vi "VNA test.vi"() -> ()   [LabVIEW 2022 SP3, in "Agilent ENA Series.lvlib"]
uses:
  <instrlib>/Agilent ENA Series/Agilent ENA Series.lvlib
  <vilib>/Utility/file.llb/Write Delimited Spreadsheet (DBL).vi
panel:
  in  "Number of Measurement Points (201)":i32=201
  in  "file path (dialog if empty) 2":path
  out "source":string
  in  "Measurement Parameter (0:S11)":u16(ring) items=["S11", "S21", "S31", "S41", "S12", "S22", "S32", "S42", "S13", "S23", "S33", "S43", "S14", "S24", "S34", "S44", "A", "B", "C", "D", "R1", "R2", "R3", "R4", "AUX1", "AUX2", "TR", "T", "R"]
  out "Waveform Graph":dbl[](graph)
  in  "VISA resource name":refnum<visa-resource-name>
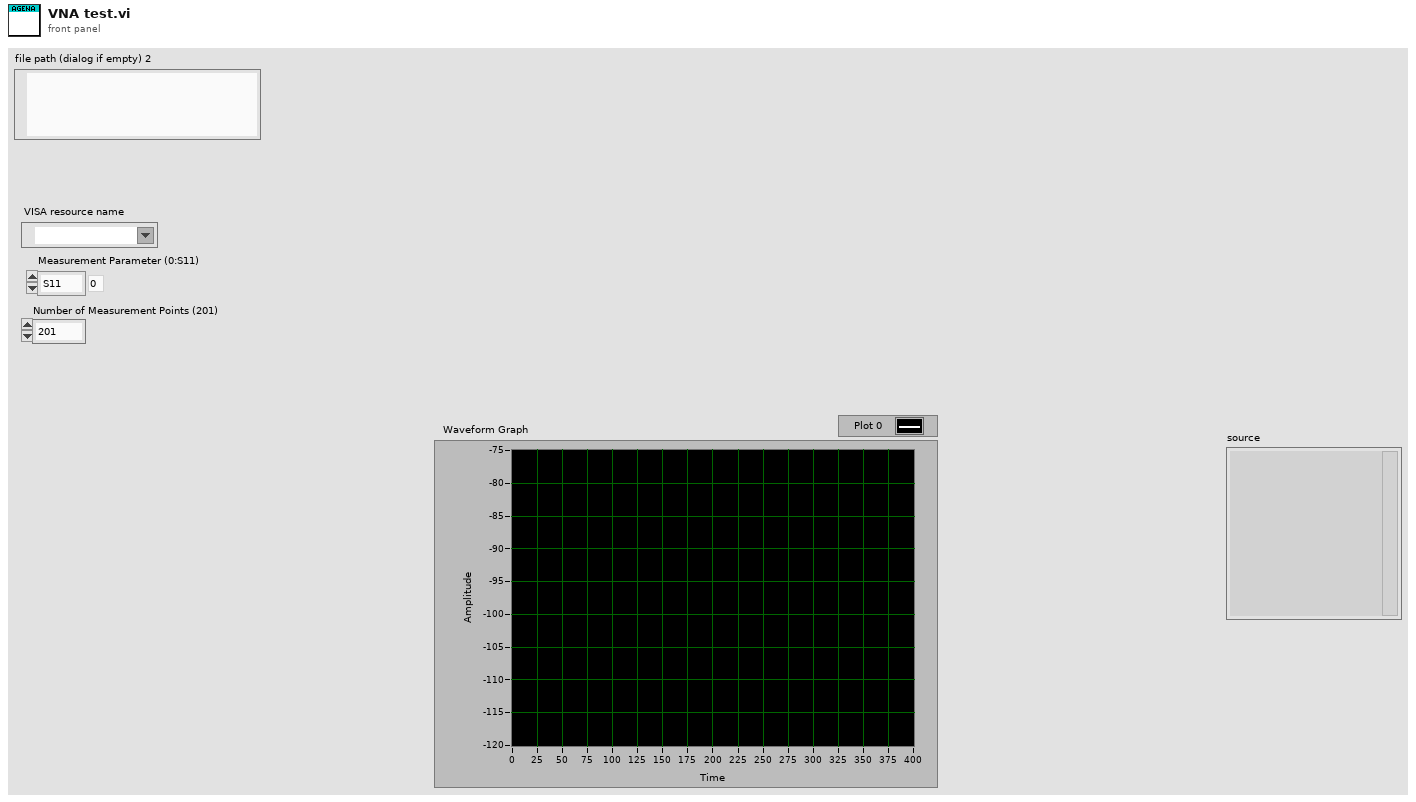
[diagram p1: front panel]
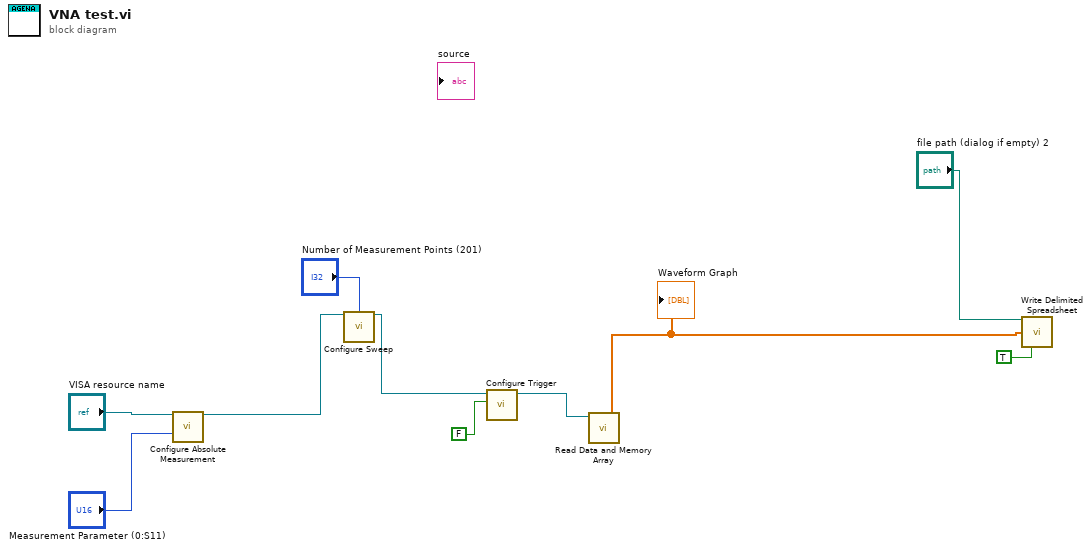
[diagram p0: block diagram]
diagram:
  n1 = call <instrlib>:"Configure Absolute Measurement.vi"("VISA resource name"="VISA resource name", "Measurement Parameter (0:S11)"="Measurement Parameter (0:S11)") -> ("VISA resource name out"=w3:refnum<visa-resource-name>)  [unwired: 12 in, 1 out]
  n2 = call <instrlib>:"Configure Sweep.vi"("VISA resource name"=w3, "Number of Measurement Points (201)"="Number of Measurement Points (201)") -> ("VISA resource name out"=w2:refnum<visa-resource-name>)  [unwired: 12 in, 1 out]
  n3 = call <instrlib>:"Configure Trigger.vi"("Continuous Sweep (T: Enable)"=FALSE, "VISA resource name"=w2) -> ("VISA resource name out"=w10:refnum<visa-resource-name>)  [unwired: 8 in, 1 out]
  n4 = call <instrlib>:"Read Data and Memory Array.vi"("VISA resource name"=w10) -> ("Primary / Real"=w5:dbl[])  [unwired: 7 in, 3 out]
  "Waveform Graph" <- w5
  n5 = call-poly <vilib>:"Write Delimited Spreadsheet.vi"("file path (dialog if empty)"="file path (dialog if empty) 2", "1D data"=w5, "transpose? (no:F)"=TRUE) -> ()  [unwired: 11 in, 2 out]
